vi "receive channel names.vi"(10 "Cluster in":T1, 11 "data":variant) -> (3 "Cluster out":T1)   [LabVIEW 2018]
uses:
  custom sub vis/speedlineData.ctl
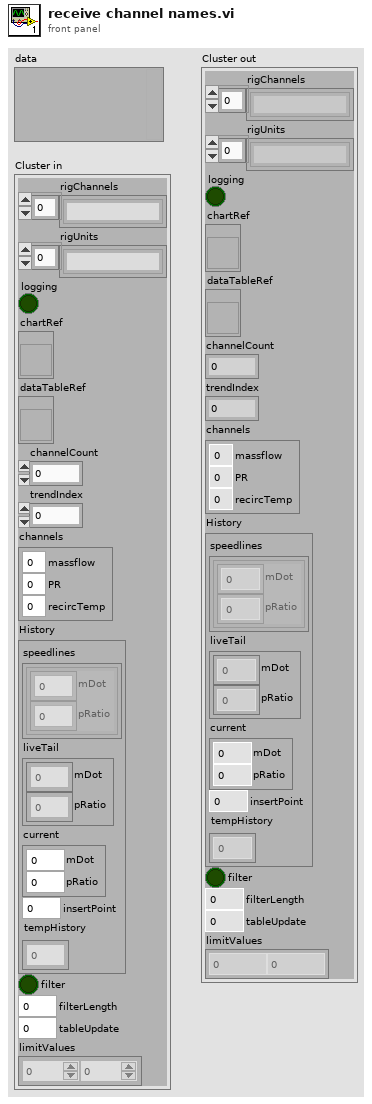
[diagram p1: front panel]
types:
  T1 = typedef "speedlineData.ctl" = cluster{"rigChannels":string[], "rigUnits":string[], "logging":bool, "chartRef":refnum<vi>, "dataTableRef":refnum<vi>, "channelCount":i32, "trendIndex":i32, "channels":cluster{"massflow":i32, "PR":i32, "recircTemp":i32}, "History":cluster{"speedlines":cluster{"mDot":dbl[], "pRatio":dbl[]}[], "liveTail":cluster{"mDot":dbl[], "pRatio":dbl[]}, "current":cluster{"mDot":dbl, "pRatio":dbl}, "insertPoint":i32, "tempHistory":dbl[][]}, "filter":bool, "filterLength":i32, "tableUpdate":i16, "limitValues":dbl[][]}
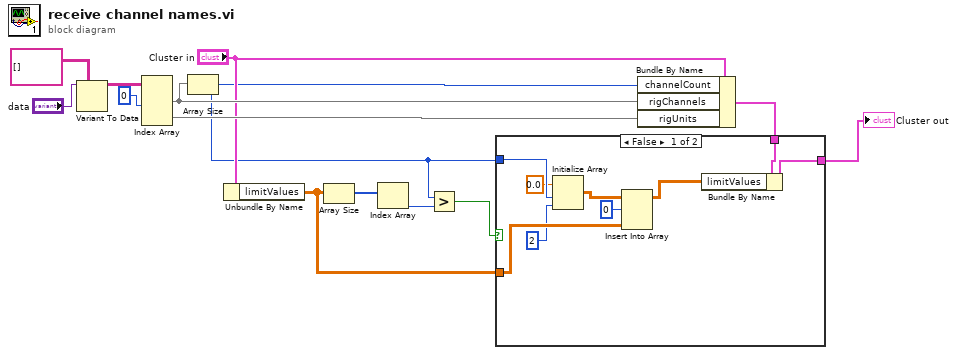
[diagram p0: block diagram]
diagram:
  n1 = Variant To Data(type=string[][] [], Variant="data") -> (data=w11:string[][])  [unwired: 1 in, 1 out]
  n2 = Index Array(array=w11, index (col) #1=0 ("index (row)")) -> (element #1=w14:string[], element #2=w10:string[])  [unwired: 3 in]
  n3 = Array Size(array=w14) -> (size(s)=w2:i32)
  n4 = Unbundle By Name("Cluster in") -> ("limitValues"=w1:dbl[][])
  n5 = Array Size(array=w1) -> (size(s)=w7:i32[])
  n6 = Index Array(array=w7) -> (element=w6:i32)  [unwired: 1 in]
  n7 = Greater?(x=w2, y=w6) -> (0:w5:bool)
  n8 = Bundle By Name(cluster="Cluster in", "channelCount"=w2, "rigChannels"=w14, "rigUnits"=w10) -> (w3:T1)
  n9 = case shown="False" w5 {
    tunnel: [w22 w24] -> w4
    tunnel: w3 -> [w23 w24]
    tunnel: w2 -> [w20 _]
    tunnel: w1 -> [w21 _]
    frame False {
      n10 = Initialize Array(0.0 ("element"), w20, 2 ("disabled index (col)")) -> (w18:dbl[][])
      n11 = Insert Into Array(array=w18, index (row)=0, new element=w21) -> (w15:dbl[][])  [unwired: 1 in]
      n12 = Bundle By Name(cluster=w23, "limitValues"=w15) -> (w22:T1)
    }
    frame True {
    }
  }
  "Cluster out" <- w4
